vi "Build Unicode Phrase.vi"(0 "PDF Report IN":refnum<class "PDF Report Class.lvclass">, 11 "error in (no error)":errorcluster) -> (4 "PDF Report OUT":refnum<class "PDF Report Class.lvclass">, 15 "error out":errorcluster)   [LabVIEW 2019]
doc: "Version 1.1\nDeveloped by Jean-Marc Simard\nCopyright © 2012, Exaprom Inc.\nAll rights reserved.\nLicense: BSD\n\nWith iTextSharp 4.1.6 (http://itextsharp.sourceforge.net)\nunder Mozilla Public License Version 1.1\n(http://www.mozilla.org/MPL/MPL-1.1.html)"
uses:
  C:/Program Files/National Instruments/LabVIEW 2019/user.lib/Exaprom PDF/DLL/itextsharp.dll
  DLL/itextsharp.dll
  <userlib>/Exaprom PDF/LV Class/PDF Report Class/PDF Report Class.lvclass
panel:
  in  "Boolean":bool
  out "Phrase":refnum<k24>
  in  "Unicode String":string
  in  "Font":refnum<k24>
  in  "leading":sgl
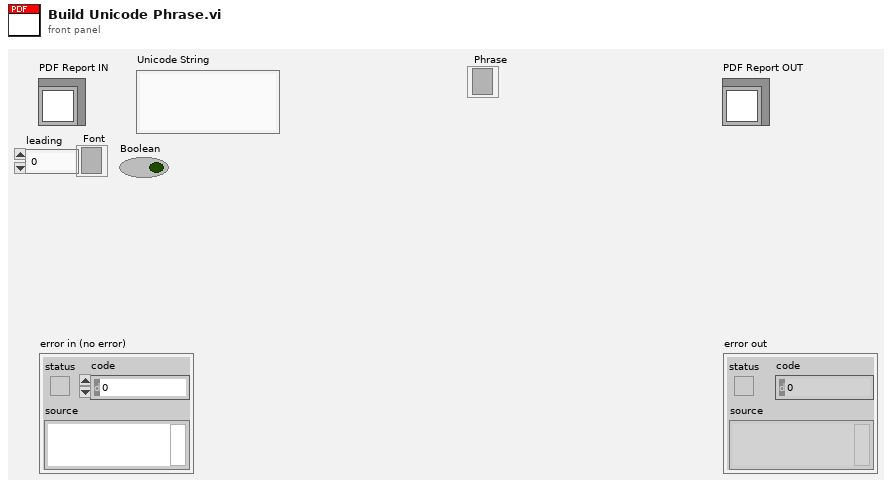
[diagram p1: front panel]
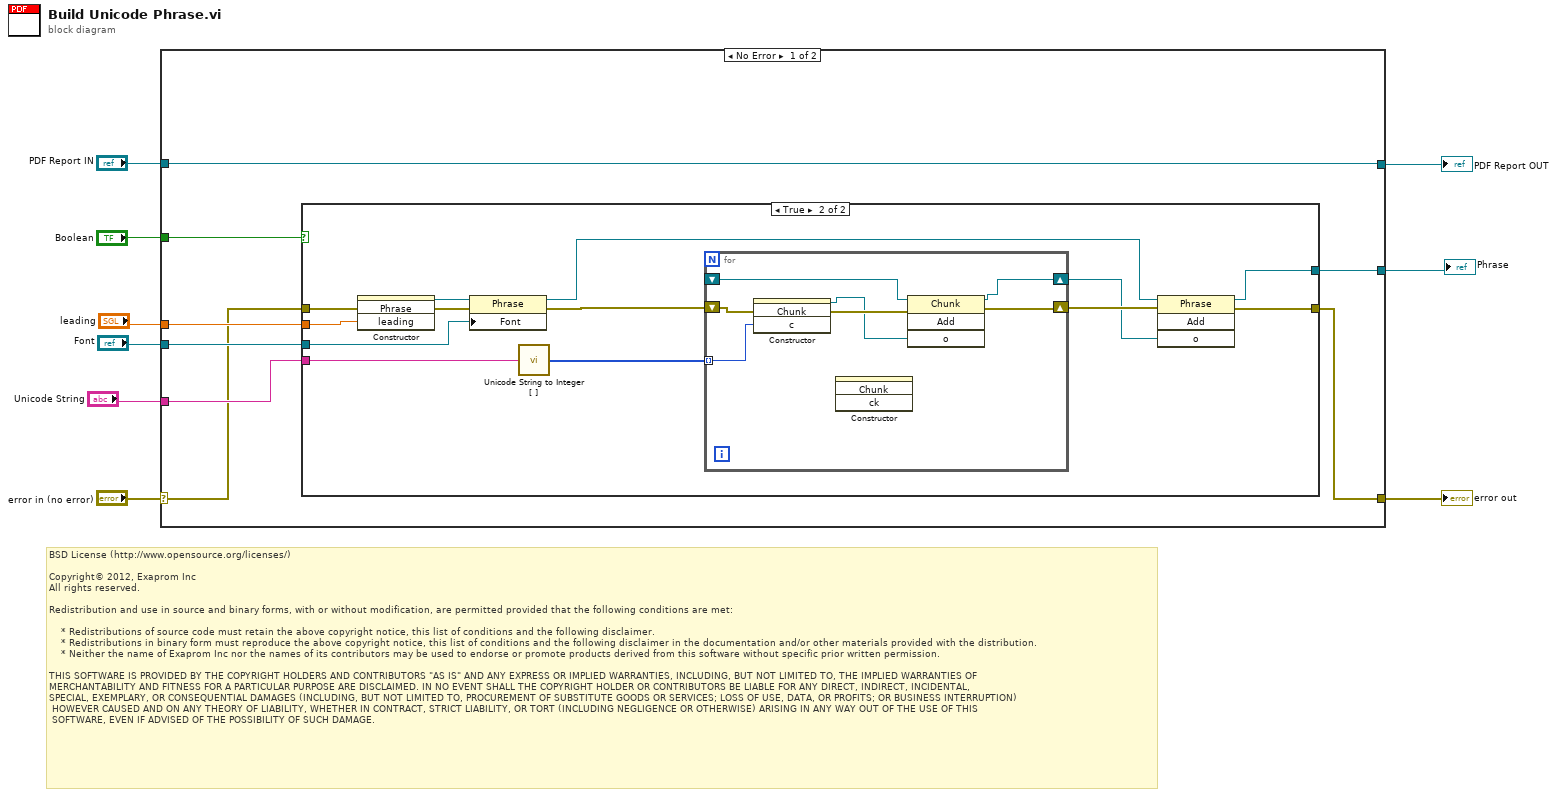
[diagram p0: block diagram]
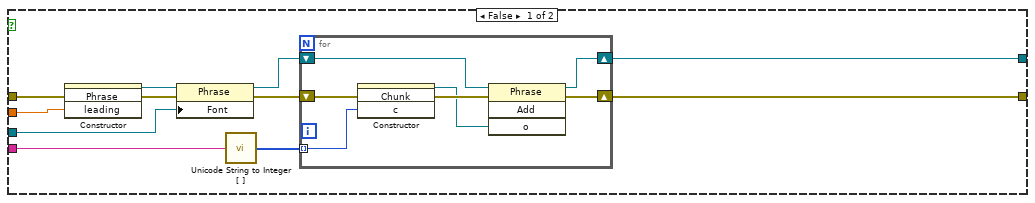
[diagram p2: hidden frame]
diagram:
  # "BSD License (http://www.opensource.org/licenses/)\n\nCopyright© 2012, Exaprom Inc\nAll rights reserved.\n\nRedistribution and use in source and binary forms, with or without modification, are permitted provided that the following conditions are met:\n\n    * Redistributions of source code must retain the above copyright notice, this list of conditions and the following disclaimer.\n    * Redistributions in binary form must reproduce the above copyright notice, this list of conditions and the following disclaimer in the documentation and/or other materials provided with the distribution.\n    * Neither the name of Exaprom Inc nor the names of its contributors may be used to endorse or promote products derived from this software without specific prior written permission.\n\nTHIS SOFTWARE IS PROVIDED BY THE COPYRIGHT HOLDERS AND CONTRIBUTORS \"AS IS\" AND ANY EXPRESS OR IMPLIED WARRANTIES, INCLUDING, BUT NOT LIMITED TO, THE IMPLIED WARRANTIES OF \nMERCHANTABILITY AND FITNESS FOR A PARTICULAR PURPOSE ARE DISCLAIMED. IN NO EVENT SHALL THE COPYRIGHT HOLDER OR CONTRIBUTORS BE LIABLE FOR ANY DIRECT, INDIRECT, INCIDENTAL,\nSPECIAL, EXEMPLARY, OR CONSEQUENTIAL DAMAGES (INCLUDING, BUT NOT LIMITED TO, PROCUREMENT OF SUBSTITUTE GOODS OR SERVICES; LOSS OF USE, DATA, OR PROFITS; OR BUSINESS INTERRUPTION)\n HOWEVER CAUSED AND ON ANY THEORY OF LIABILITY, WHETHER IN CONTRACT, STRICT LIABILITY, OR TORT (INCLUDING NEGLIGENCE OR OTHERWISE) ARISING IN ANY WAY OUT OF THE USE OF THIS\n SOFTWARE, EVEN IF ADVISED OF THE POSSIBILITY OF SUCH DAMAGE."
  n1 = case shown="No Error" "error in (no error)" {
    selector: "error in (no error)" -> [w11 w57]
    tunnel: "PDF Report IN" -> [w17 w56]
    tunnel: [w17 w56] -> w8
    tunnel: [w12 w57] -> w7
    tunnel: "leading" -> [w16 _]
    tunnel: "Font" -> [w15 _]
    tunnel: "Unicode String" -> [w14 _]
    tunnel: [w13 _] -> w2
    tunnel: "Boolean" -> [w10 _]
    frame No Error {
      n2 = case shown="True" w10 {
        tunnel: w16 -> [w23 w45]
        tunnel: w15 -> [w22 w44]
        tunnel: w14 -> [w21 w43]
        tunnel: [w20 w42] -> w13
        tunnel: [w19 w41] -> w12
        tunnel: w11 -> [w18 w40]
        frame False {
          n3 = constructor class="Phrase"(error in=w18, "leading"=w23) -> (reference out=w26:refnum<k24>, error out=w28:errorcluster)  [unwired: 2 in, 2 out]
          n4 = property class="Phrase"(reference=w26, error in=w28, "Font"=w22) -> (reference out=w25:refnum<k24>, error out=w27:errorcluster)
          n5 = call <userlib>:"Unicode String to Integer [ ].vi"("Unicode String"=w21) -> ("Char U16 [ ]"=w24:u16[])  [unwired: 12 in, 2 out]
          n6 = for {
            tunnel: w24 -> [w35] mode=indexing
            shift-right: [w31] -> w20
            shift-left: w25 -> [w34]
            shift-right: [w29] -> w19
            shift-left: w27 -> [w30]
            n7 = constructor class="Chunk"(error in=w30, "c"=w35) -> (reference out=w32:refnum<k24>, error out=w33:errorcluster)  [unwired: 2 in, 2 out]
            n8 = invoke class="Phrase" method="Add"(reference=w34, error in=w33, "o"=w32) -> (reference out=w31:refnum<k24>, error out=w29:errorcluster)  [unwired: 1 in, 2 out]
          }
        }
        frame True {
          n9 = constructor class="Phrase"(error in=w40, "leading"=w45) -> (reference out=w47:refnum<k24>, error out=w48:errorcluster)  [unwired: 2 in, 2 out]
          n10 = property class="Phrase"(reference=w47, error in=w48, "Font"=w44) -> (reference out=w46:refnum<k24>, error out=w36:errorcluster)
          n11 = call <userlib>:"Unicode String to Integer [ ].vi"("Unicode String"=w43) -> ("Char U16 [ ]"=w39:u16[])  [unwired: 12 in, 2 out]
          n12 = for {
            shift-right: [w55] -> w38
            shift-left: w36 -> [w52]
            shift-right: [w53] -> w37
            shift-left: _ -> [w54]
            tunnel: w39 -> [w49] mode=indexing
            n13 = constructor class="Chunk"(error in=w52, "c"=w49) -> (reference out=w50:refnum<k24>, error out=w51:errorcluster)  [unwired: 2 in, 2 out]
            n14 = constructor class="Chunk"() -> ()  [unwired: 4 in, 4 out]
            n15 = invoke class="Chunk" method="Add"(reference=w54, error in=w51, "o"=w50) -> (reference out=w53:refnum<k24>, error out=w55:errorcluster)  [unwired: 1 in, 2 out]
          }
          n16 = invoke class="Phrase" method="Add"(reference=w46, error in=w38, "o"=w37) -> (reference out=w42:refnum<k24>, error out=w41:errorcluster)  [unwired: 1 in, 2 out]
        }
      }
    }
    frame Error {
    }
  }
  "PDF Report OUT" <- w8
  "error out" <- w7
  "Phrase" <- w2
